vi "VI Springboard.vi"() -> ()   [LabVIEW 2016]
panel:
  out "Individual Classes":string[](array[string])
  out "Common Class":string
  in  "ACTION":bool
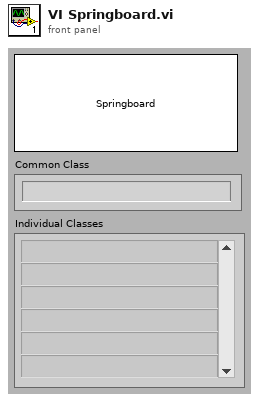
[diagram p1: front panel]
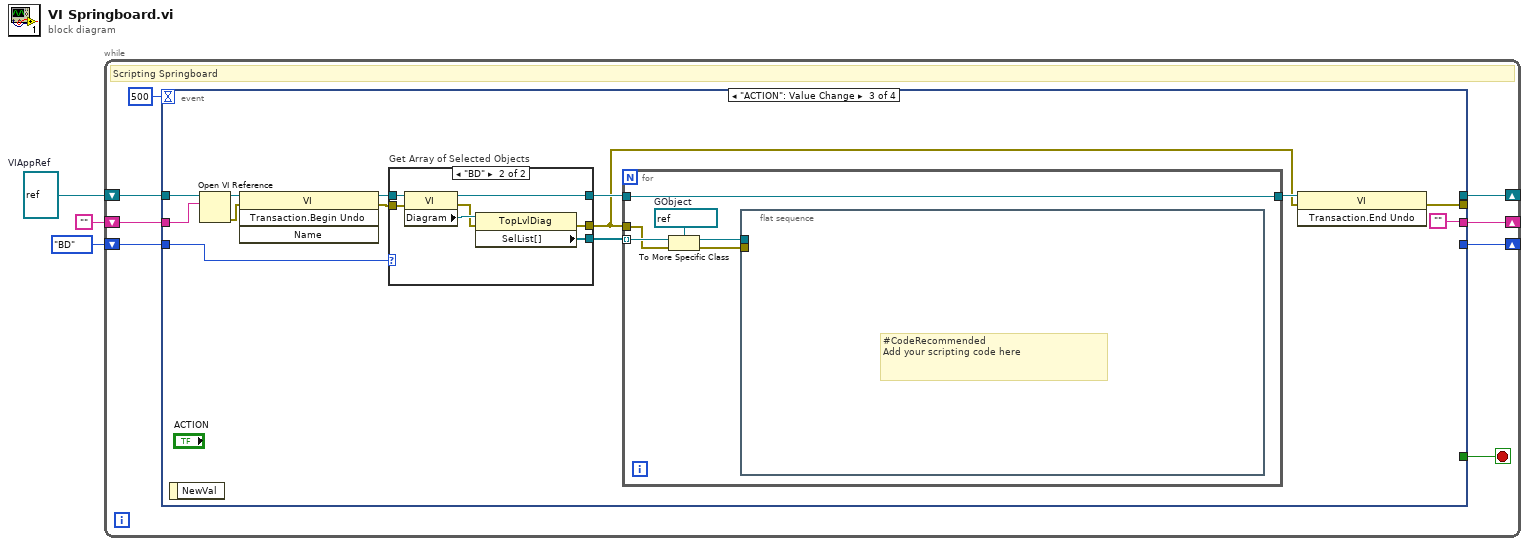
[diagram p0: block diagram]
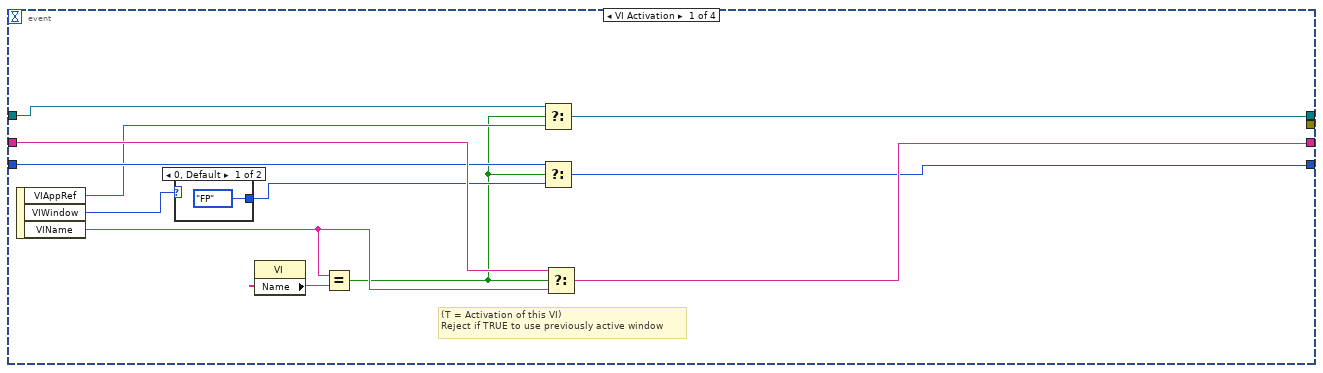
[diagram p2: hidden frame]
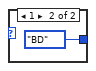
[diagram p3: hidden frame]
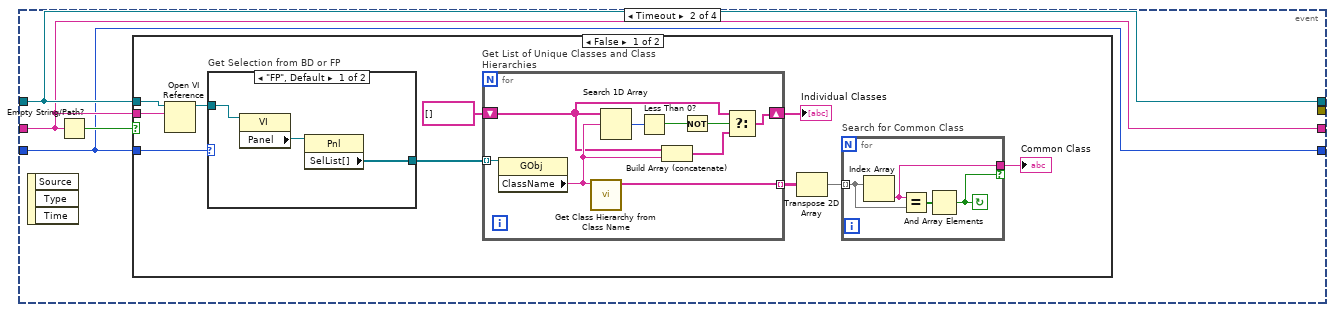
[diagram p4: hidden frame]
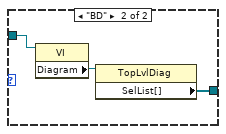
[diagram p5: hidden frame]
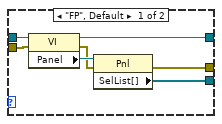
[diagram p7: hidden frame]
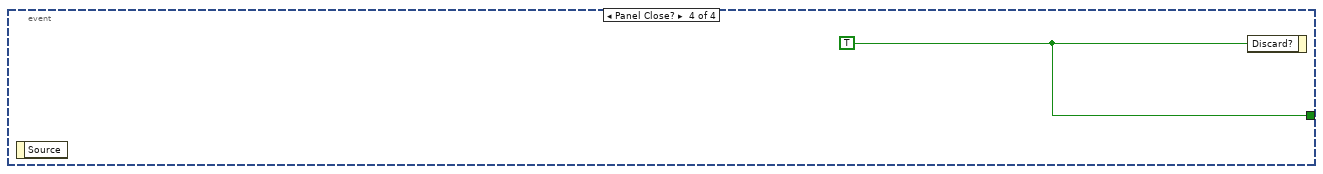
[diagram p8: hidden frame]
diagram:
  w1 = refnum<vi> refnum  # VIAppRef
  n1 = while {
    shift-right: [w11] -> _
    shift-left: "" -> [w10]
    shift-right: [w8] -> _
    shift-left: enum16{"FP", "BD"}."BD" -> [w7]
    shift-right: [w6] -> _
    shift-left: w1 -> [w5]
    stop <- w9 stop-if-true
    # "Scripting Springboard"
    n2 = event shown="[2] \"ACTION\": Value Change" {
      selector: _ -> [_ _ _ _]
      dyn-events: _ -> [_ _ _ _]
      timeout: 500 -> [_ _ _ _]
      tunnel: [w20 w27 "" _] -> w11
      tunnel: w10 -> [w23 w27 w71 _]
      tunnel: [_ _ _ w92] -> w9
      tunnel: [w18 w26 _ _] -> w8
      tunnel: w7 -> [w19 w26 w69 _]
      tunnel: [w14 w28 _ _] -> w6
      tunnel: w5 -> [w13 w28 w70 _]
      tunnel: [_ _ w60 _] -> _
      event VI Activation {
        # "(T = Activation of this VI)\nReject if TRUE to use previously active window"
        n3 = event-data() -> ("VIAppRef"=w15:refnum<vi>, "VIWindow"=w17:i32, "VIName"=w21:string)  [unwired: 1 out]
        n4 = case shown="0, Default" w17 {
          tunnel: [enum16{"FP", "BD"}."FP" enum16{"FP", "BD"}."BD"] -> w16
          frame 0, Default {
          }
          frame 1 {
          }
        }
        n5 = property class="VI"() -> ("Name"=w22:string)  [unwired: 2 in, 2 out]
        n6 = Equal?(x=w21, y=w22) -> (x = y?=w12:bool)
        n7 = Select(t=w13, s=w12, f=w15) -> (s? t:f=w14:refnum<vi>)
        n8 = Select(t=w19, s=w12, f=w16) -> (s? t:f=w18:enum16{"FP", "BD"})
        n9 = Select(t=w23, s=w12, f=w21) -> (s? t:f=w20:string)
      }
      event Timeout {
        n10 = event-data() -> ()  [unwired: 4 out]
        n11 = Empty String/Path?(string/path=w27) -> (empty?=w29:bool)
        n12 = case shown="False" w29 {
          tunnel: w28 -> [w39 _]
          tunnel: w27 -> [w38 _]
          tunnel: w26 -> [w36 _]
          frame False {
            n13 = Open VI Reference(application reference (local)=w39, vi path=w38) -> (vi reference=w37:refnum<vi>)  [unwired: 4 in, 1 out]
            n14 = case "Get Selection from BD or FP" shown="\"FP\", Default" w36 {
              tunnel: w37 -> [w54 w57]
              tunnel: [w53 w56] -> w35
              frame "FP", Default {
                n15 = property class="VI"(reference=w54) -> ("Panel"=w55:refnum<vi>)  [unwired: 1 in, 2 out]
                n16 = property class="Pnl"(reference=w55) -> ("SelList[]"=w53:refnum<vi>[])  [unwired: 1 in, 2 out]
              }
              frame "BD" {
                n17 = property class="VI"(reference=w57) -> ("Diagram"=w58:refnum<vi>)  [unwired: 1 in, 2 out]
                n18 = property class="TopLvlDiag"(reference=w58) -> ("SelList[]"=w56:refnum<vi>[])  [unwired: 1 in, 2 out]
              }
            }
            n19 = for "Get List of Unique Classes and Class Hierarchies" {
              tunnel: w35 -> [w52] mode=indexing
              shift-right: [w45] -> w33
              shift-left: string[] [] -> [w46]
              tunnel: [w44] -> w32 mode=indexing
              n20 = property class="GObj"(reference=w52) -> ("ClassName"=w49:string)  [unwired: 1 in, 2 out]
              n21 = call <vilib>:"Get Class Hierarchy from Class Name.vi"("Class Name"=w49) -> ("Class Hierarchy"=w44:string[])  [unwired: 9 in, 1 out]
              n22 = Search 1D Array(1D array=w46, element=w49) -> (index of element=w51:i32)  [unwired: 1 in]
              n23 = Less Than 0?(x=w51) -> (x < 0?=w50:bool)
              n24 = Build Array (concatenate)(w46, w49) -> (w47:string[])
              n25 = Not(x=w50) -> (.not. x?=w48:bool)
              n26 = Select(t=w46, s=w48, f=w47) -> (s? t:f=w45:string[])
            }
            "Individual Classes" <- w33
            n27 = Transpose 2D Array(2D array=w32) -> (transposed array=w30:string[][])
            n28 = for "Search for Common Class" {
              tunnel: w30 -> [w43] mode=indexing
              tunnel: [w41] -> w31 if=w40
              stop <- w40 continue-if-true
              n29 = Index Array(array=w43) -> (element=w41:string)  [unwired: 1 in]
              n30 = Equal?(x=w41, y=w43) -> (x = y?=w42:bool[])
              n31 = And Array Elements(Boolean array=w42) -> (logical AND=w40:bool)
            }
            "Common Class" <- w31
          }
          frame True {
          }
        }
      }
      event "ACTION": Value Change {
        n32 = event-data() -> ()  [unwired: 2 out]
        n33 = Open VI Reference(application reference (local)=w70, vi path=w71) -> (vi reference=w68:refnum<vi>, error out=w63:errorcluster)  [unwired: 2 in, 2 out]
        n34 = invoke class="VI" method="Transaction.Begin Undo"(reference=w68, error in=w63) -> (reference out=w66:refnum<vi>, error out=w62:errorcluster)  [unwired: 2 in, 2 out]
        n35 = case "Get Array of Selected Objects" shown="\"BD\"" w69 {
          tunnel: w66 -> [w83 w90]
          tunnel: [w82 w89] -> w67
          tunnel: [w81 w88] -> w64
          tunnel: w62 -> [w80 w87]
          tunnel: [w78 w85] -> w59
          frame "FP", Default {
            n36 = property class="VI"(reference=w83, error in=w80) -> (reference out=w81:refnum<vi>, error out=w79:errorcluster, "Panel"=w84:refnum<vi>)
            n37 = property class="Pnl"(reference=w84, error in=w79) -> (error out=w78:errorcluster, "SelList[]"=w82:refnum<vi>[])  [unwired: 1 out]
          }
          frame "BD" {
            n38 = property class="VI"(reference=w90, error in=w87) -> (reference out=w88:refnum<vi>, error out=w86:errorcluster, "Diagram"=w91:refnum<vi>)
            n39 = property class="TopLvlDiag"(reference=w91, error in=w86) -> (error out=w85:errorcluster, "SelList[]"=w89:refnum<vi>[])  [unwired: 1 out]
          }
        }
        n40 = for {
          tunnel: w67 -> [w76] mode=indexing
          tunnel: [w77] -> w65
          tunnel: w64 -> [w77]
          tunnel: w59 -> [w75]
          w74 = refnum<vi> refnum  # GObject
          n41 = To More Specific Class(target class=w74, reference=w76, error in=w75) -> (specific class reference=w73:refnum<vi>, error out=w72:errorcluster)
          n42 = flat-sequence {
            tunnel: w73 -> [_]
            tunnel: w72 -> [_]
            frame #0 {
              # "#CodeRecommended\nAdd your scripting code here"
            }
          }
        }
        n43 = invoke class="VI" method="Transaction.End Undo"(reference=w65, error in=w59) -> (error out=w60:errorcluster)  [unwired: 1 in, 2 out]
      }
      event Panel Close? {
        w92 = TRUE ("Discard?")
        n44 = event-data() -> ()  [unwired: 2 out]
        n45 = event-data("Discard?"=w92) -> ()  [unwired: 1 in, 1 out]
      }
    }
  }
